vi "Calibrate Acceleration 2 Ticks (uSMC).vi"(1 "Acceleration Value":dbl) -> (0 "Acceleration ticks":u8)   [LabVIEW 2010, in "SignalWriterMH110203USBStepperMotor.lvclass"]
uses:
  SignalWriterMH110203USBStepperMotor.lvclass
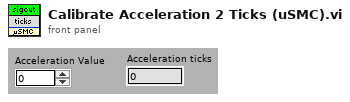
[diagram p1: front panel]
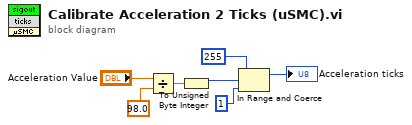
[diagram p0: block diagram]
diagram:
  n1 = Divide(x="Acceleration Value", y=98.0) -> (x/y=w6:dbl)
  n2 = To Unsigned Byte Integer(number=w6) -> (unsigned 8bit integer=w7:u8)
  n3 = In Range and Coerce(upper limit=u8 255, x=w7, lower limit=u8 1) -> (coerced(x)=→"Acceleration ticks":u8)  [unwired: 1 out]
